vi "Main.vi"(11 "Module Admin":refnum<class "Delacor_lib_QMH_Module Admin.lvclass">) -> ()   [LabVIEW 2023, in "Adjust FP VIs.lvlib"]
doc: "This template is based off of the Queued Message Handler design pattern and the Queued Message Handler project template that ships with LabVIEW.\n\nThe main difference is that the queue is private to this module and communication between modules is performed via Broadcast and Request events.\n\nRequest events are wrapped in public API methods and are handled in the Event Handling Loop (EHL) of this VI. Any module can register for Broadcast events sent by this module. The EHL generates messages based on user interface actions.\n\nThe Message Handling Loop (MHL) processes messages generated by the EHL, or by other messages. The messages are string values, so new messages can be added easily to the Message Cases case structure in the MHL. Each message cluster can also provide an optional value for Message Data, which is a variant that can be converted to whatever message-specific data is required.\n_____\nBased on DQMH Dev Tools: Project Template 7.1.2.1547."
uses:
  Adjust FP VIs.lvlib
  <vilib>/Delacor/Delacor QMH/Libraries/Module Admin_class/Delacor_lib_QMH_Module Admin.lvclass
  Module Data--cluster.ctl
  Stop Argument--cluster.ctl
  <vilib>/Delacor/Delacor QMH/Libraries/Message Queue_class/Delacor_lib_QMH_Message Queue.lvclass/Delacor_lib_QMH_Message Queue.ctl
  <vilib>/Delacor/Delacor QMH/Libraries/Module Admin_class/Delacor_lib_QMH_Module Admin.lvclass/Delacor_lib_QMH_Module Admin.ctl
  <vilib>/Utility/miscctls.llb/LVPointTypeDef.ctl
  <vilib>/Delacor/Delacor QMH/Libraries/Message Queue_class/Delacor_lib_QMH_Enqueue Message (Single).vi
  <vilib>/Delacor/Delacor QMH/Libraries/Module Admin_class/Delacor_lib_QMH_Get External Launch.vi
  <vilib>/Delacor/Delacor QMH/Libraries/Message Queue_class/Delacor_lib_QMH_Message Queue.lvclass
panel:
  in  "OK Button":bool
  in  "Project Path":path
  out "Total VIs to Adjust":i32
  out "Front Panels Adjusted":u8(slide) scale=0.0..100.0
  out "error out":errorcluster
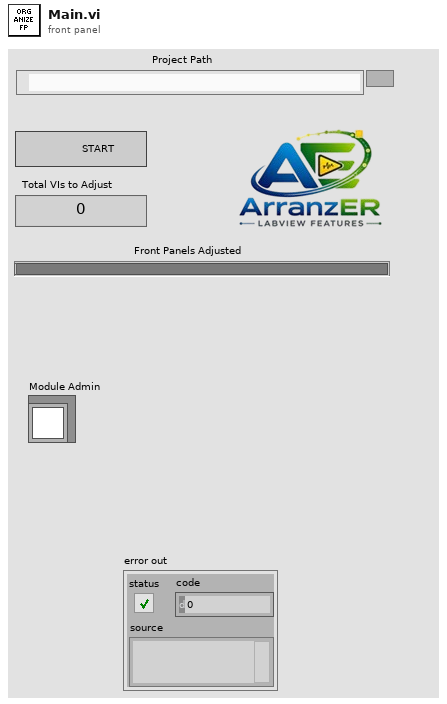
[diagram p1: front panel]
types:
  T1 = typedef "Adjust FP VIs.lvlib/Request Events--cluster.ctl" = cluster{"Stop Module":refnum<user-event>, "Show Panel":refnum<user-event>, "Hide Panel":refnum<user-event>, "Get Module Execution Status":refnum<user-event>, "Show Diagram":refnum<user-event>, "Private.Adjust FP for VIs":refnum<user-event>}
  T2 = typedef "Adjust FP VIs.lvlib/Module Data--cluster.ctl" = cluster{"Status":string, "VIs Name":string[], "VI Ref":refnum<vi>[], "Project Path":path, "Project:Open":refnum<vi>}
  T3 = typedef "LVPointTypeDef.ctl" = cluster{"Horizontal":i16, "Vertical":i16}
  T4 = enum32{"Invalid", "Standard", "Closed", "Hidden", "Minimized", "Maximized"}
  T5 = typedef "Adjust FP VIs.lvlib/Stop Argument--cluster.ctl" = cluster{"Origin":string, "Exit via Stop Module Req?":bool, "Wait for Module to stop?":bool}
  T6 = enum32{"invalid lock state", "Not Locked", "Locked (No Password)", "Password-protected"}
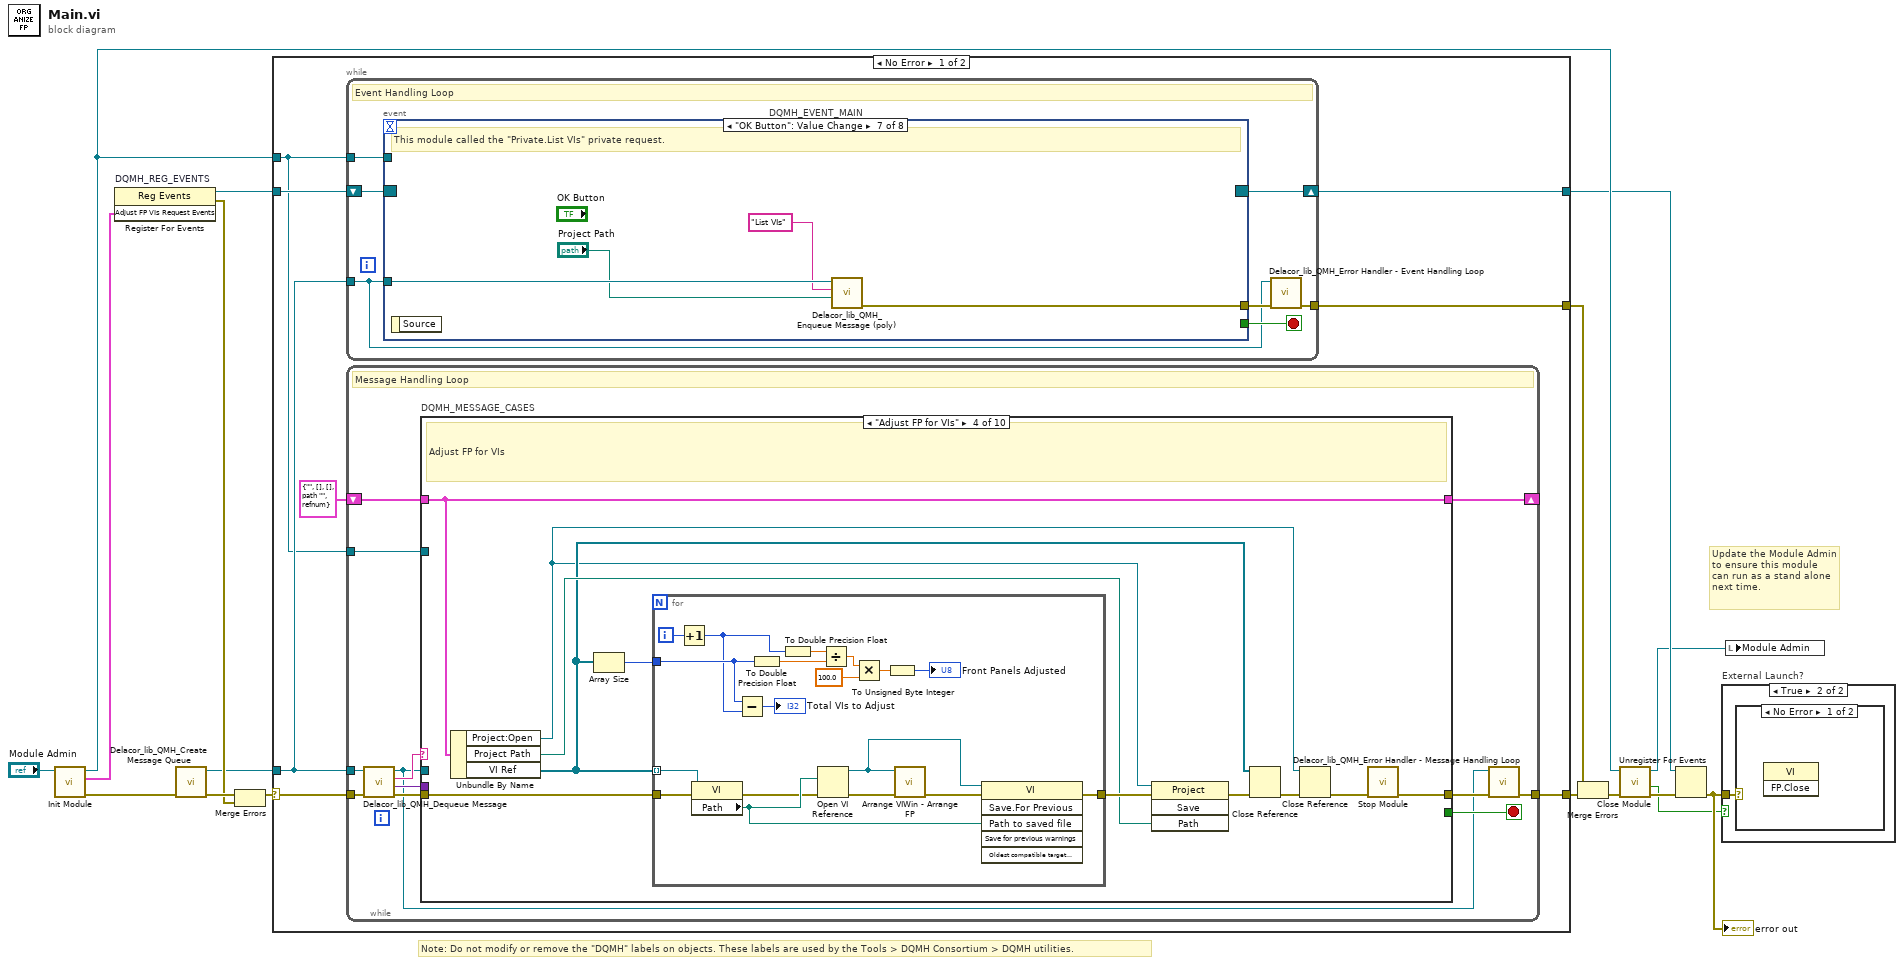
[diagram p0: block diagram]
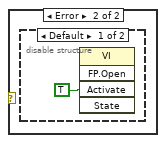
[diagram p3: hidden frame]
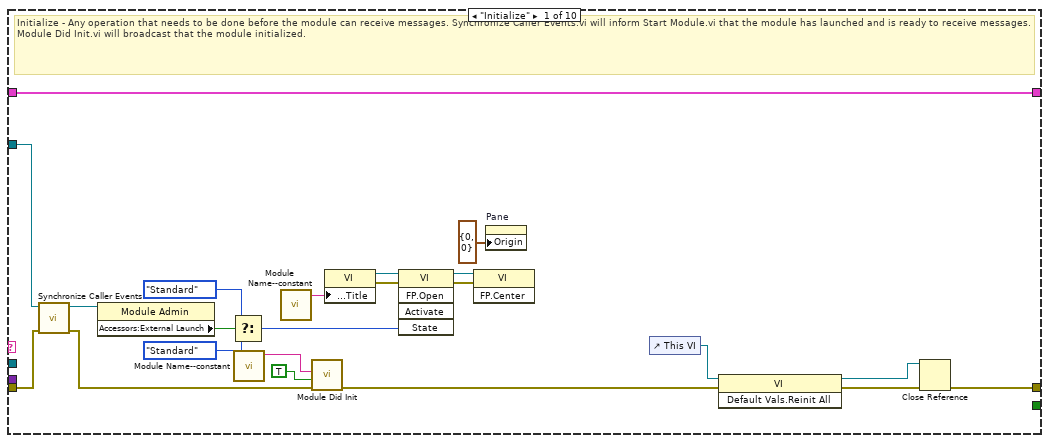
[diagram p5: hidden frame]
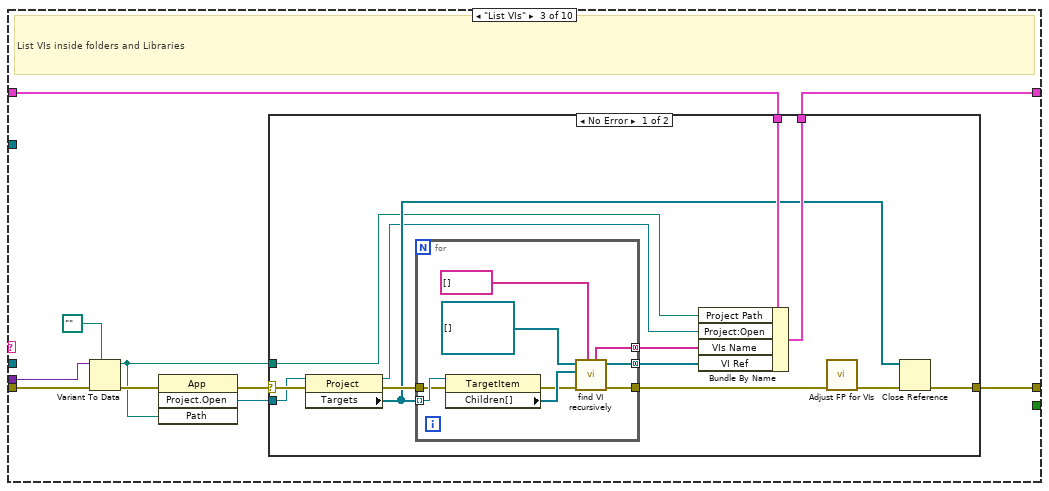
[diagram p7: hidden frame]
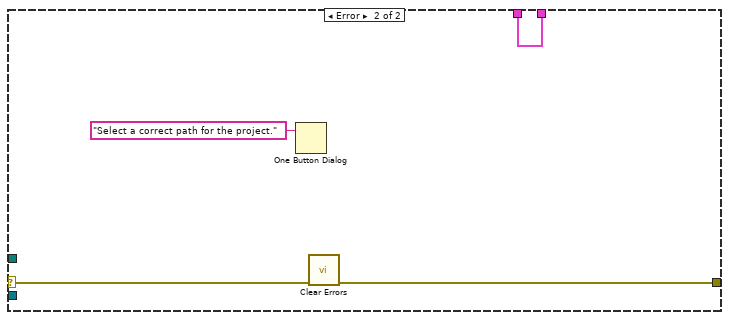
[diagram p8: hidden frame]
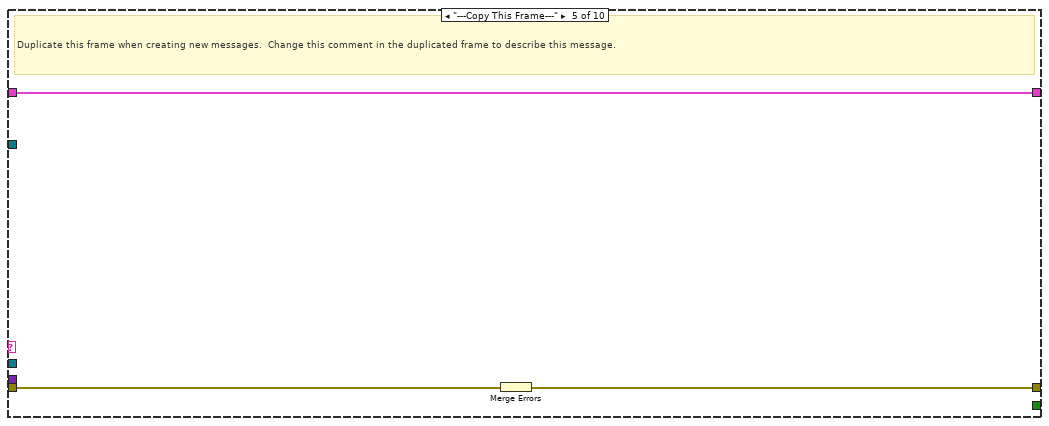
[diagram p9: hidden frame]
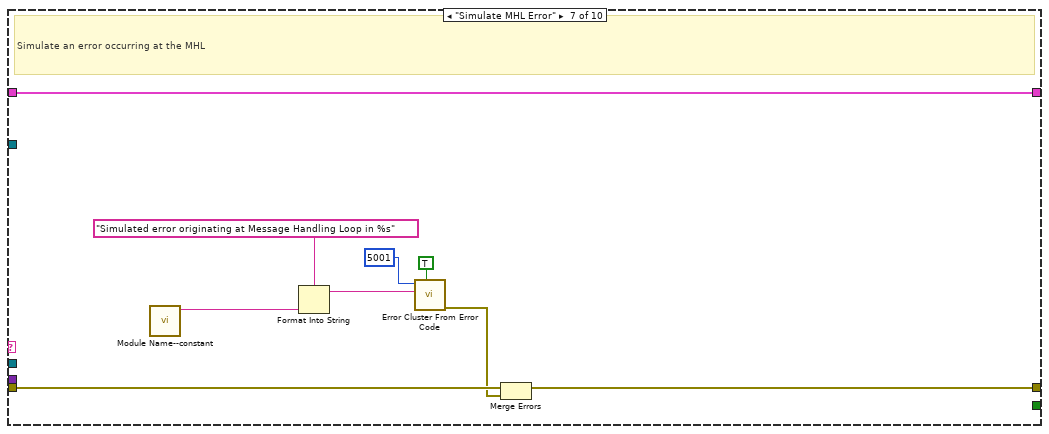
[diagram p11: hidden frame]
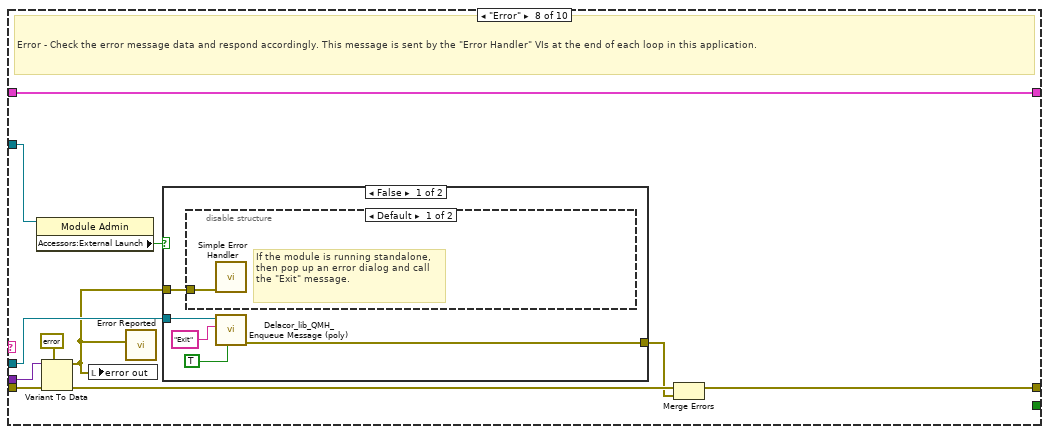
[diagram p12: hidden frame]
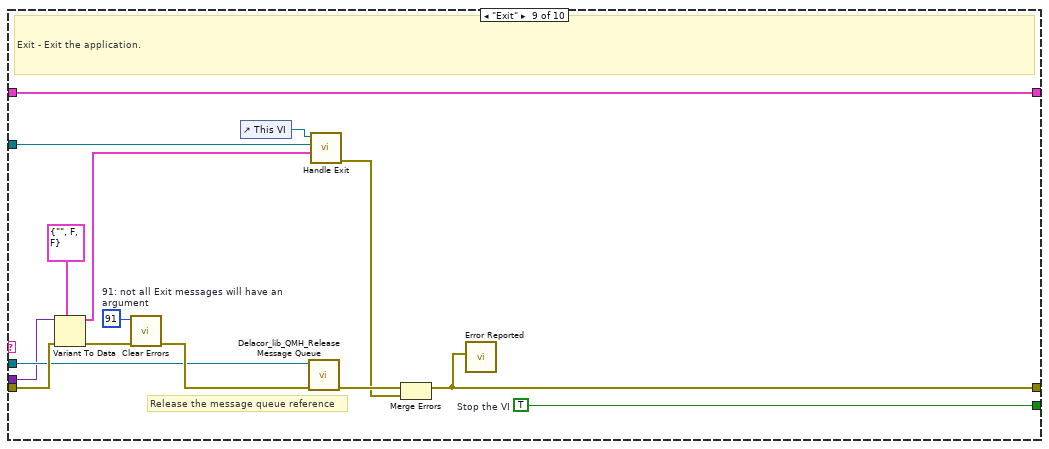
[diagram p15: hidden frame]
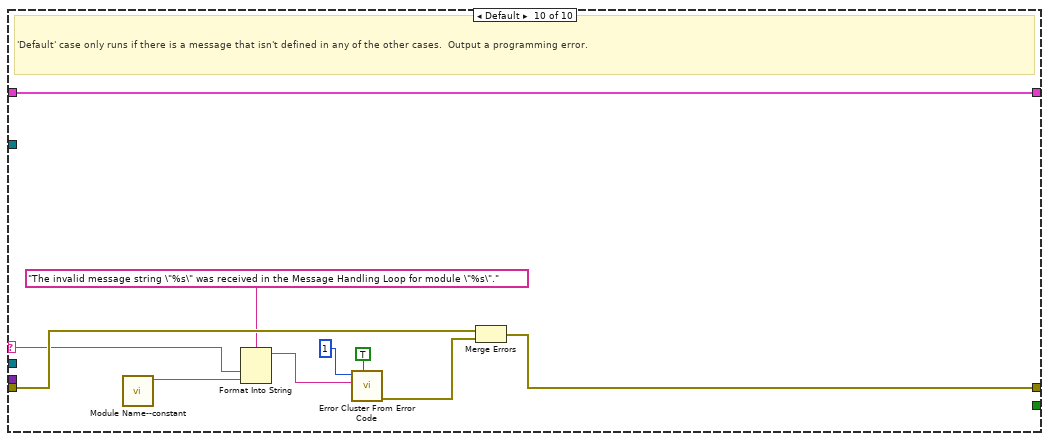
[diagram p16: hidden frame]
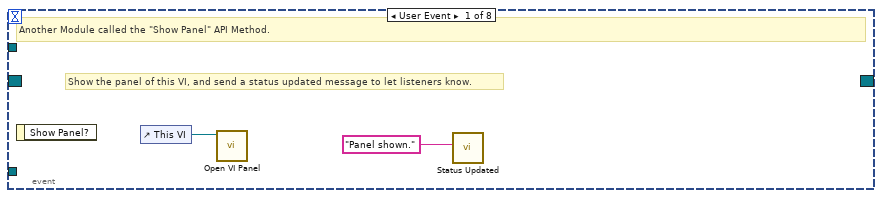
[diagram p17: hidden frame]
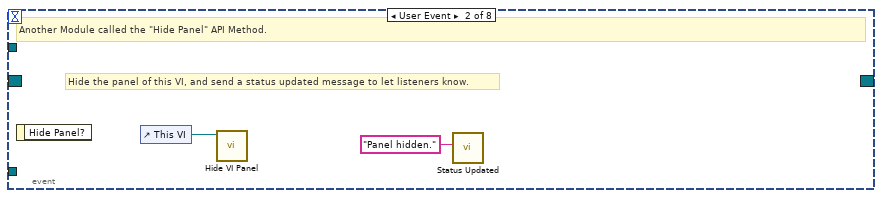
[diagram p18: hidden frame]
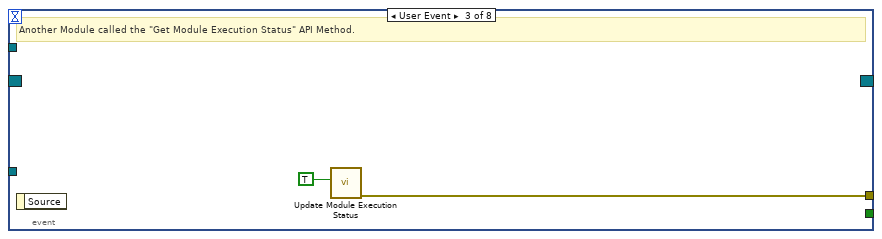
[diagram p19: hidden frame]
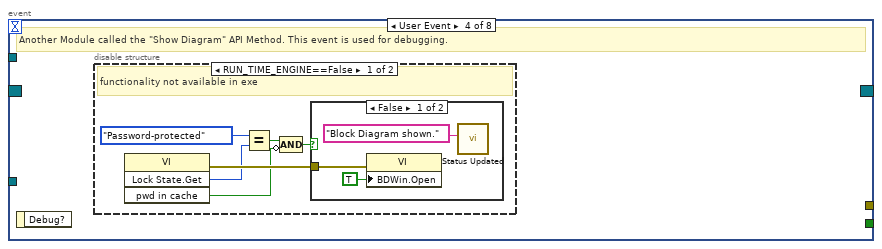
[diagram p20: hidden frame]
diagram:
  # "Note: Do not modify or remove the \"DQMH\" labels on objects. These labels are used by the Tools > DQMH Consortium > DQMH utilities."
  # "Update the Module Admin to ensure this module can run as a stand alone next time."
  n1 = call "Init Module.vi"("Singleton Module Admin in"="Module Admin") -> ("error out"=w16:errorcluster, "Adjust FP VIs Request Events"=w5:T1, "Singleton Module Admin out"=w8:refnum<class "Delacor_lib_QMH_Module Admin.lvclass">)  [unwired: 8 in]
  n2 = register-events "DQMH_REG_EVENTS"(w5) -> (reference out=w6:refnum<event-registration>, error out=w9:errorcluster)  [unwired: 2 in]
  n3 = call <vilib>:"Delacor_lib_QMH_Create Message Queue.vi"("error in"=w16) -> ("error out"=w11:errorcluster, "Message Queue"=w4:refnum<class "Delacor_lib_QMH_Message Queue.lvclass">)  [unwired: 9 in]
  n4 = Merge Errors(w11, w9) -> (w10:errorcluster)
  n5 = case shown="No Error" w10 {
    selector: w10 -> [w23 w242]
    tunnel: [w25 w241] -> w17
    tunnel: [w22 w240] -> w7
    tunnel: w6 -> [w20 w240]
    tunnel: w4 -> [w19 w235]
    tunnel: [w24 _] -> w14
    tunnel: w8 -> [w18 w236]
    frame No Error {
      n6 = while {
        tunnel: w19 -> [w183]
        shift-right: [w186] -> w22
        shift-left: w20 -> [w187]
        tunnel: [w188] -> w24
        tunnel: w18 -> [w184]
        stop <- w185 stop-if-true
        # "Event Handling Loop"
        n7 = event "DQMH_EVENT_MAIN" shown="[6] \"OK Button\": Value Change" {
          selector: w187 -> [_ _ _ _ _ _ _ _]
          dyn-events: [_ _ _ _ _ _ _ _] -> w186
          timeout: _ -> [_ _ _ _ _ _ _ _]
          tunnel: [_ _ _ _ TRUE ("Discard?") _ _ _] -> w185
          tunnel: w183 -> [_ _ _ _ w211 w218 w231 w234]
          tunnel: [_ _ w195 _ w214 w220 w229 w232] -> w189
          tunnel: w184 -> [_ _ _ _ _ w217 _ _]
          event User Event {
            # "Show the panel of this VI, and send a status updated message to let listeners know."
            # "Another Module called the \"Show Panel\" API Method."
            n8 = event-data() -> ()  [unwired: 1 in, 1 out]
            n9 = control-ref of="This VI"() -> (w191:refnum<vi>)
            n10 = call "Open VI Panel.vi"("VI"=w191) -> ()  [unwired: 10 in, 1 out]
            n11 = call "Status Updated.vi"("Status"="Panel shown." ("format string")) -> ()  [unwired: 10 in, 1 out]
          }
          event User Event {
            # "Hide the panel of this VI, and send a status updated message to let listeners know."
            # "Another Module called the \"Hide Panel\" API Method."
            n12 = event-data() -> ()  [unwired: 1 in, 1 out]
            n13 = control-ref of="This VI"() -> (w193:refnum<vi>)
            n14 = call "Hide VI Panel.vi"("VI"=w193) -> ()  [unwired: 10 in, 1 out]
            n15 = call "Status Updated.vi"("Status"="Panel hidden." ("format string")) -> ()  [unwired: 10 in, 1 out]
          }
          event User Event {
            # "Another Module called the \"Get Module Execution Status\" API Method."
            n16 = event-data() -> ()  [unwired: 1 in, 1 out]
            n17 = call "Update Module Execution Status.vi"("Running?"=TRUE) -> ("error out"=w195:errorcluster)  [unwired: 10 in]
          }
          event User Event {
            # "Another Module called the \"Show Diagram\" API Method. This event is used for debugging."
            n18 = event-data() -> ()  [unwired: 1 in, 1 out]
            n19 = disable-structure shown="RUN_TIME_ENGINE==False" {
              frame condition #0 (active) {
                # "functionality not available in exe"
                n20 = invoke on="Invoke Node" class="VI" method="Lock State.Get"() -> (error out=w201:errorcluster, "Get Lock State"=w200:T6, "pwd in cache"=w197:bool)  [unwired: 4 in, 1 out]
                n21 = Equal?(x=T6."Password-protected", y=w200) -> (x = y?=w198:bool)
                n22 = Compound Arithmetic op=AND(w198, invert w197) -> (w196:bool)
                n23 = case shown="False" w196 {
                  tunnel: w201 -> [w204 _]
                  frame False {
                    n24 = property on="Property Node" class="VI"(error in=w204, "BDWin.Open"=TRUE ("Block Diagram Window:Open")) -> ()  [unwired: 1 in, 2 out]
                    n25 = call "Status Updated.vi"("Status"="Block Diagram shown." ("format string")) -> ()  [unwired: 10 in, 1 out]
                  }
                  frame True {
                    # "Password-protected VI, and the password is not in the cache. Do not show the diagram."
                  }
                }
              }
              frame condition #1 {
              }
            }
          }
          event User Event {
            # "The Stop Module Event can get fired from the Exit message in the MHL. The queue gets destroyed in that case. If the queue no longer exists, the Enqueue Exit as a priority message will return error 1. It is safe to ignore, because the module is already exiting."
            # "Another Module called the \"Stop Module\" API Method  or the Message Handling Loop below."
            n26 = event-data() -> ("Exit via Stop Module Req?"=w207:bool, "Wait for Module to stop?"=w206:bool)  [unwired: 1 in]
            n27 = Bundle By Name(cluster=T5 {"Origin"="", "Exit via Stop Module Req?"=FALSE, "Wait for Module to stop?"=FALSE} ("Stop Argument"), "Exit via Stop Module Req?"=w207, "Wait for Module to stop?"=w206) -> (w205:T5)
            n28 = call-poly <vilib>:"Delacor_lib_QMH_Enqueue Message (poly).vi"("Priority Message? (F)"=TRUE, "Message Data"=w205, "Message"="Exit", "Message Queue in"=w211) -> ("error out"=w215:errorcluster)  [unwired: 6 in, 1 out]
            n29 = call <vilib>:"Clear Errors.vi"("error in (no error)"=w215, "specific error code to clear (0: all)"=1) -> ("error out"=w214:errorcluster)  [unwired: 4 in, 1 out]
          }
          event Panel Close? {
            w219 = TRUE  # Discard the event, the MHL is responsible for closing and stopping this VI.
            # "Hide the panel or send the 'Exit' message if the user clicks the 'X' on the module main VI panel."
            n30 = event-data() -> ()  [unwired: 1 in, 1 out]
            n31 = property on="Property Node" class="Module Admin"(reference=w217) -> ("Accessors:External Launch"=w216:bool)  [unwired: 1 in, 2 out]
            n32 = case shown="False" w216 {
              tunnel: w218 -> [_ w226]
              tunnel: [_ w227] -> w220
              frame True {
                # "If externally launched, clicking the 'X' hides the panel, but doesn't close it."
                n33 = control-ref of="This VI"() -> (w223:refnum<vi>)
                n34 = call "Hide VI Panel.vi"("VI"=w223) -> ("error out"=w221:errorcluster)  [unwired: 10 in]
                n35 = call "Status Updated.vi"("error in"=w221, "Status"="Panel hidden." ("format string")) -> ()  [unwired: 9 in, 1 out]
              }
              frame False {
                # "If run as a stand-alone VI, clicking the panel 'X' stops the VI."
                n36 = call-poly <vilib>:"Delacor_lib_QMH_Enqueue Message (poly).vi"("Priority Message? (F)"=TRUE, "Message"="Exit", "Message Queue in"=w226) -> ("error out"=w227:errorcluster)  [unwired: 7 in, 1 out]
              }
            }
            n37 = event-data ("Event Filter Node")("Discard?"=w219) -> ()  [unwired: 1 in, 1 out]
          }
          event "OK Button": Value Change {
            # "This module called the \"Private.List VIs\" private request."
            n38 = event-data() -> ()  [unwired: 1 in, 1 out]
            n39 = call-poly <vilib>:"Delacor_lib_QMH_Enqueue Message (poly).vi"("Message Data"="Project Path", "Message"="List VIs", "Message Queue in"=w231) -> ("error out"=w229:errorcluster)  [unwired: 7 in, 1 out]
          }
          event User Event {
            # "This module called the \"Private.Adjust FP for VIs\" private request."
            n40 = event-data() -> ()  [unwired: 1 in, 1 out]
            n41 = call-poly <vilib>:"Delacor_lib_QMH_Enqueue Message (poly).vi"("Message"="Adjust FP for VIs", "Message Queue in"=w234) -> ("error out"=w232:errorcluster)  [unwired: 8 in, 1 out]
          }
        }
        n42 = call-dynamic "Delacor_lib_QMH_Error Handler - Event Handling Loop.vi"("error in"=w189, "Message Queue in"=w183) -> ("dup error in"=w188:errorcluster)  [unwired: 8 in, 1 out]
      }
      n43 = while {
        tunnel: w19 -> [w26]
        shift-right: [w34] -> _
        shift-left: T2 {"Status"="", "VIs Name"=[], "VI Ref"=[], "Project Path"=path "", "Project:Open"=refnum} ("Data Cluster") -> [w35]
        tunnel: w23 -> [w37]
        tunnel: [w29] -> w25
        tunnel: w18 -> [w30]
        stop <- w33 stop-if-true
        # "Message Handling Loop"
        n44 = call-dynamic "Delacor_lib_QMH_Dequeue Message.vi"("error in"=w37, "Message Queue in"=w26) -> ("error out"=w36:errorcluster, "Message Data"=w31:variant, "Message"=w32:string, "Message Queue out"=w27:refnum<class "Delacor_lib_QMH_Message Queue.lvclass">)  [unwired: 6 in]
        n45 = case "DQMH_MESSAGE_CASES" shown="\"Adjust FP for VIs\"" w32 {
          selector: w32 -> [_ _ _ _ _ _ _ _ _ w178]
          tunnel: w27 -> [_ _ _ _ _ _ _ w144 w166 _]
          tunnel: w36 -> [w57 w61 w68 w108 w129 w131 w140 w151 w172 w181]
          tunnel: [w40 w61 w69 w98 w128 w131 w139 w147 w167 w182] -> w28
          tunnel: w35 -> [w47 w60 w70 w107 w127 w130 w137 w146 w158 w179]
          tunnel: [w47 w60 w71 w107 w127 w130 w137 w146 w158 w179] -> w34
          tunnel: [_ _ _ _ _ _ _ _ w165 _] -> w33
          tunnel: w31 -> [_ _ w63 _ _ _ _ w145 w164 _]
          tunnel: w30 -> [w48 _ _ _ _ _ _ w143 w159 _]
          frame "Initialize" {
            # "Initialize - Any operation that needs to be done before the module can receive messages. Synchronize Caller Events.vi will inform Start Module.vi that the module has launched and is ready to receive messages. Module Did Init.vi will broadcast that the module initialized."
            n46 = call "Synchronize Caller Events.vi"("error in"=w57, "Singleton Module Admin in"=w48) -> ("error out"=w56:errorcluster, "Singleton Module Admin out"=w44:refnum<class "Delacor_lib_QMH_Module Admin.lvclass">)  [unwired: 8 in]
            n47 = property on="Property Node" class="Module Admin"(reference=w44) -> ("Accessors:External Launch"=w52:bool)  [unwired: 1 in, 2 out]
            n48 = Select(t=T4."Standard" ("State"), s=w52, f=T4."Standard" ("State")) -> (s? t:f=w49:T4)
            n49 = call "Module Name--constant.vi"() -> ("Module Name"=w45:string)  [unwired: 11 in]
            n50 = call "Module Name--constant.vi"() -> ("Module Name"=w55:string)  [unwired: 11 in]
            n51 = call "Module Did Init.vi"("error in"=w56, "Initialized?"=TRUE, "Origin"=w45) -> ("error out"=w38:errorcluster)  [unwired: 8 in]
            n52 = property on="Property Node" class="VI"("Front Panel.Title"=w55) -> (reference out=w54:refnum<vi>, error out=w59:errorcluster)  [unwired: 2 in]
            n53 = invoke on="Invoke Node" class="VI" method="FP.Open"(reference=w54, error in=w59, "State"=w49) -> (reference out=w53:refnum<vi>, error out=w58:errorcluster)  [unwired: 2 in, 3 out]
            n54 = invoke on="Invoke Node" class="VI" method="FP.Center"(reference=w53, error in=w58) -> ()  [unwired: 1 in, 3 out]
            n55 = property on="Pane" class="Pane"("Origin"=T3 {"Horizontal"=0, "Vertical"=0}) -> ()  [unwired: 2 in, 2 out]
            n56 = control-ref of="This VI"() -> (w41:refnum<vi>)
            n57 = invoke class="VI" method="Default Vals.Reinit All"(reference=w41, error in=w38) -> (reference out=w39:refnum<vi>, error out=w42:errorcluster)  [unwired: 1 in, 1 out]
            n58 = Close Reference(reference=w39, error in (no error)=w42) -> (error out=w40:errorcluster)
          }
          frame "---Module Specific---" {
            # "Separator -- The following cases handle messages specific to this Module."
          }
          frame "List VIs" {
            # "List VIs inside folders and Libraries"
            n59 = Variant To Data(error in=w68, type=path "", Variant=w63) -> (data=w62:path, error out=w65:errorcluster)
            n60 = invoke class="App" method="Project.Open"(error in=w65, "Path"=w62) -> (error out=w66:errorcluster, "Project:Open"=w67:refnum<vi>)  [unwired: 2 in, 2 out]
            n61 = case shown="No Error" w66 {
              selector: w66 -> [w77 w97]
              tunnel: [w81 w96] -> w71
              tunnel: w70 -> [w80 w96]
              tunnel: [w76 w94] -> w69
              tunnel: w67 -> [w74 _]
              tunnel: w62 -> [w73 _]
              frame No Error {
                n62 = property on="Property Node" class="Project"(reference=w74, error in=w77) -> (reference out=w72:refnum<vi>, error out=w84:errorcluster, "Targets"=w75:refnum<vi>[])
                n63 = for {
                  tunnel: w75 -> [w93] mode=indexing
                  tunnel: w84 -> [w92]
                  tunnel: [w87] -> w79
                  tunnel: [w86] -> w82 mode=concatenating
                  tunnel: [w85] -> w83 mode=concatenating
                  n64 = property on="Property Node" class="TargetItem"(reference=w93, error in=w92) -> (error out=w89:errorcluster, "Children[]"=w90:refnum<vi>[])  [unwired: 1 out]
                  n65 = call "find VI recursively.vi"("VIs Name"=string[] [], "error in (no error)"=w89, "Project Item"=w90, "VI Ref In"=refnum<vi>[] [] ("Array")) -> ("error out"=w87:errorcluster, "VI Ref Out"=w86:refnum<vi>[], "VIs Name Out"=w85:string[])  [unwired: 5 in]
                }
                n66 = Bundle By Name(cluster=w80, "Project Path"=w73, "Project:Open"=w72, "VIs Name"=w83, "VI Ref"=w82) -> (w81:T2)
                n67 = call "Adjust FP for VIs.vi"("error in"=w79) -> ("error out"=w78:errorcluster)  [unwired: 10 in]
                n68 = Close Reference(reference=w75, error in (no error)=w78) -> (error out=w76:errorcluster)
              }
              frame Error {
                n69 = One Button Dialog(message="Select a correct path for the project.") -> ()  [unwired: 1 in, 1 out]
                n70 = call <vilib>:"Clear Errors.vi"("error in (no error)"=w97) -> ("error out"=w94:errorcluster)  [unwired: 5 in, 1 out]
              }
            }
          }
          frame "Adjust FP for VIs" {
            # "Adjust FP for VIs"
            n71 = Unbundle By Name(w107) -> ("Project:Open"=w100:refnum<vi>, "Project Path"=w104:path, "VI Ref"=w101:refnum<vi>[])
            n72 = Array Size(array=w101) -> (size(s)=w106:i32)
            n73 = for {
              tunnel: w108 -> [w118]
              tunnel: [w117] -> w105
              tunnel: w101 -> [w119] mode=indexing
              tunnel: w106 -> [w110]
              i -> [w126]
              n74 = Increment(x=w126) -> (x+1=w109:i32)
              n75 = property class="VI"(reference=w119, error in=w118) -> (error out=w113:errorcluster, "Path"=w116:path)  [unwired: 1 out]
              n76 = Subtract(x=w110, y=w109) -> (x-y=→"Total VIs to Adjust":i32)
              n77 = To Double Precision Float(number=w110) -> (double precision float=w124:dbl)
              n78 = To Double Precision Float(number=w109) -> (double precision float=w125:dbl)
              n79 = Open VI Reference(vi path=w116, error in (no error)=w113) -> (vi reference=w112:refnum<vi>, error out=w115:errorcluster)  [unwired: 4 in]
              n80 = Divide(x=w125, y=w124) -> (x/y=w123:dbl)
              n81 = Multiply(x=w123, y=100.0) -> (x*y=w121:dbl)
              n82 = To Unsigned Byte Integer(number=w121) -> (unsigned 8bit integer=→"Front Panels Adjusted":u8)
              n83 = call <resource>:"Arrange VIWin - Arrange FP.vi"("VI"=w112, "error in"=w115) -> ("error out"=w114:errorcluster)  [unwired: 13 in]
              n84 = invoke class="VI" method="Save.For Previous"(reference=w112, error in=w114, "Path to saved file"=w116) -> (error out=w117:errorcluster)  [unwired: 3 in, 5 out]
            }
            n85 = invoke class="Project" method="Save"(reference=w100, error in=w105, "Path"=w104) -> (error out=w102:errorcluster)  [unwired: 1 in, 3 out]
            n86 = Close Reference(reference=w101, error in (no error)=w102) -> (error out=w103:errorcluster)
            n87 = Close Reference(reference=w100, error in (no error)=w103) -> (error out=w99:errorcluster)
            n88 = call "Stop Module.vi"("error in"=w99) -> ("error out"=w98:errorcluster)  [unwired: 10 in]
          }
          frame "---Copy This Frame---" {
            # "Duplicate this frame when creating new messages.  Change this comment in the duplicated frame to describe this message."
            n89 = Merge Errors(w129) -> (w128:errorcluster)
          }
          frame "---Exit and Error Handling---" {
            # "Separator - The following cases handle errors and exit messages."
          }
          frame "Simulate MHL Error" {
            # "Simulate an error occurring at the MHL"
            n90 = call "Module Name--constant.vi"() -> ("Module Name"=w133:string)  [unwired: 11 in]
            n91 = Format Into String(format string="Simulated error originating at Message Handling Loop in %s", w133) -> (resulting string=w134:string)  [unwired: 2 in, 1 out]
            n92 = call <vilib>:"Error Cluster From Error Code.vi"("show call chain? (False)"=TRUE, "error message (\"\")"=w134, "error code (0)"=5001) -> ("error out"=w138:errorcluster)  [unwired: 6 in]
            n93 = Merge Errors(w140, w138) -> (w139:errorcluster)
          }
          frame "Error" {
            # "Error - Check the error message data and respond accordingly. This message is sent by the \"Error Handler\" VIs at the end of each loop in this application."
            n94 = property on="Property Node" class="Module Admin"(reference=w143) -> ("Accessors:External Launch"=w142:bool)  [unwired: 1 in, 2 out]
            n95 = Variant To Data(error in=w151, type=errorcluster {"status"=FALSE, "code"=0, "source"=""} ("error constant"), Variant=w145) -> (data=w141:errorcluster, error out=w149:errorcluster)
            n96 = local write "error out"(w141) -> ()
            n97 = call "Error Reported.vi"("Error"=w141) -> ()  [unwired: 10 in, 1 out]
            n98 = case shown="False" w142 {
              tunnel: [w156 _] -> w148
              tunnel: w144 -> [w154 _]
              tunnel: w141 -> [w155 _]
              frame False {
                n99 = disable-structure shown="Default" {
                  disable-tunnel: w155 -> [w157 _]
                  frame condition #0 (active) {
                    # "If the module is running standalone, then pop up an error dialog and call the \"Exit\" message."
                    n100 = call <vilib>:"Simple Error Handler.vi"("error in (no error)"=w157) -> ()  [unwired: 4 in, 5 out]
                  }
                  frame condition #1 {
                    # "To prevent the Simple Error Handler VI from being loaded (e.g. when deploying to a Real-Time target), add the Conditional Disable Symbol \"DQMH_Disable_SEH\" to your project and set it to TRUE."
                  }
                }
                n101 = call-poly <vilib>:"Delacor_lib_QMH_Enqueue Message (poly).vi"("Priority Message? (F)"=TRUE, "Message"="Exit", "Message Queue in"=w154) -> ("error out"=w156:errorcluster)  [unwired: 7 in, 1 out]
              }
              frame True {
                # "If the module was launched externally, calling the Error Reported broadcast VI is the only action performed by the \"Error\" message. The module's caller can then process the error appropriately."
              }
            }
            n102 = Merge Errors(w149, w148) -> (w147:errorcluster)
          }
          frame "Exit" {
            w163 = 91  # 91: not all Exit messages will have an argument
            w165 = TRUE  # Stop the VI
            # "Release the message queue reference"
            # "Exit - Exit the application."
            n103 = Variant To Data(error in=w172, type=T5 {"Origin"="", "Exit via Stop Module Req?"=FALSE, "Wait for Module to stop?"=FALSE} ("Stop Argument"), Variant=w164) -> (data=w161:T5, error out=w169:errorcluster)
            n104 = call <vilib>:"Clear Errors.vi"("error in (no error)"=w169, "specific error code to clear (0: all)"=w163) -> ("error out"=w171:errorcluster)  [unwired: 4 in, 1 out]
            n105 = control-ref of="This VI"() -> (w160:refnum<vi>)
            n106 = call-dynamic "Delacor_lib_QMH_Release Message Queue.vi"("error in"=w171, "Message Queue"=w166) -> ("error out"=w170:errorcluster)  [unwired: 9 in]
            n107 = call "Handle Exit.vi"("Stop Argument"=w161, "Admin in"=w159, "VI reference"=w160) -> ("error out"=w168:errorcluster)  [unwired: 7 in, 1 out]
            n108 = Merge Errors(w170, w168) -> (w167:errorcluster)
            n109 = call "Error Reported.vi"("Error"=w167) -> ()  [unwired: 10 in, 1 out]
          }
          frame Default {
            # "'Default' case only runs if there is a message that isn't defined in any of the other cases.  Output a programming error."
            n110 = call "Module Name--constant.vi"() -> ("Module Name"=w177:string)  [unwired: 11 in]
            n111 = Format Into String(format string="The invalid message string \"%s\" was received in the Message Handling Loop for module \"%s\".", w178, w177) -> (resulting string=w173:string)  [unwired: 2 in, 1 out]
            n112 = call <vilib>:"Error Cluster From Error Code.vi"("show call chain? (False)"=TRUE, "error message (\"\")"=w173, "error code (0)"=1) -> ("error out"=w180:errorcluster)  [unwired: 6 in]
            n113 = Merge Errors(w181, w180) -> (w182:errorcluster)
          }
        }
        n114 = call-dynamic "Delacor_lib_QMH_Error Handler - Message Handling Loop.vi"("error in"=w28, "Message Queue in"=w27) -> ("dup error in"=w29:errorcluster)  [unwired: 8 in, 1 out]
      }
    }
    frame Error {
      # "Synchronize Caller Events.vi will inform Start Module.vi that the module has launched and will let the code calling Start Module.vi register for broadcasts and would permit the caller receive the broadcast that an error occurred at launch time."
      n115 = call-dynamic "Delacor_lib_QMH_Release Message Queue.vi"("error in"=w242, "Message Queue"=w235) -> ("error out"=w241:errorcluster)  [unwired: 9 in]
      n116 = call "Synchronize Caller Events.vi"("Singleton Module Admin in"=w236) -> ("error out"=w243:errorcluster)  [unwired: 9 in, 1 out]
      n117 = call "Module Name--constant.vi"() -> ("Module Name"=w239:string)  [unwired: 11 in]
      n118 = Format Into String(format string="An error occurred during initialization. %s is no longer running.", w239) -> (resulting string=w237:string)  [unwired: 2 in, 1 out]
      n119 = Merge Errors(w241, w243) -> (w244:errorcluster)
      n120 = call "Error Reported.vi"("Additional Information"=w237, "Error"=w244) -> ()  [unwired: 9 in, 1 out]
    }
  }
  n121 = Merge Errors(w14, w17) -> (w13:errorcluster)
  n122 = call "Close Module.vi"("error in"=w13, "Module Admin in"=w8) -> ("error out"=w15:errorcluster, "External Launch"=w1:bool, "Module Admin out"=w2:refnum<class "Delacor_lib_QMH_Module Admin.lvclass">)  [unwired: 7 in]
  n123 = Unregister For Events(event registration refnum=w7, error in=w15) -> (error out=w12:errorcluster)
  "error out" <- w12
  n124 = case "External Launch?" shown="True" w1 {
    tunnel: w12 -> [_ w245]
    frame False {
    }
    frame True {
      n125 = case shown="No Error" w245 {
        frame No Error {
          n126 = invoke on="Invoke Node" class="VI" method="FP.Close"() -> ()  [unwired: 3 in, 3 out]
        }
        frame Error {
          n127 = disable-structure shown="Default" {
            frame condition #0 (active) {
              n128 = invoke class="VI" method="FP.Open"("Activate"=TRUE ("Activate?")) -> ()  [unwired: 4 in, 5 out]
            }
            frame condition #1 {
            }
          }
        }
      }
    }
  }
  n129 = local write "Module Admin"(w2) -> ()
